vi "Deinitialize.vi"(8 "error in (no error)":errorcluster, 11 "IP Connection in":refnum<class "IP Connection.lvclass">) -> (0 "error out":errorcluster)   [LabVIEW 2011, in "Tinkerforge.lvlib" / "IP Connection.lvclass"]
doc: "This VI deinitializes the <B>IP Connection</B> class object and collects the called communication worker VI and disconnects from the Brickd."
uses:
  IP Connection.lvclass
  IP Connection.lvclass/IP Connection.ctl
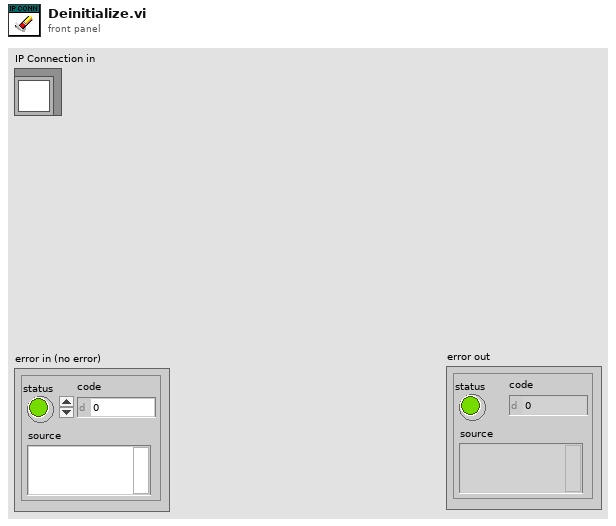
[diagram p1: front panel]
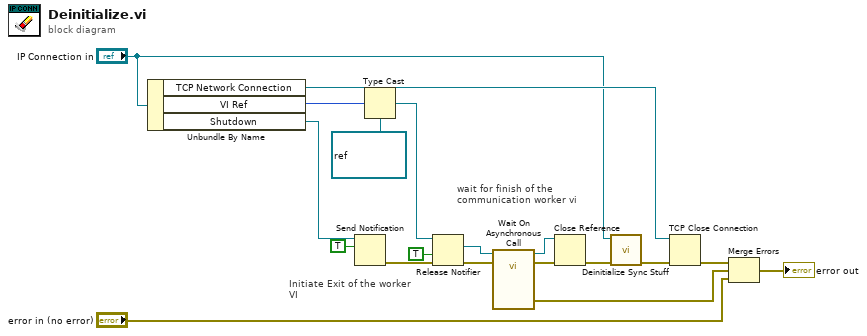
[diagram p0: block diagram]
diagram:
  # "Initiate Exit of the worker\nVI"
  # "wait for finish of the\ncommunication worker vi"
  n1 = Unbundle By Name("IP Connection in") -> ("TCP Network Connection"=w19:refnum<k5>, "VI Ref"=w18:u32, "Shutdown"=w2:refnum<notifier>)
  n2 = Send Notification(notification=TRUE, notifier=w2) -> (error out=w3:errorcluster)  [unwired: 1 in, 1 out]
  n3 = Type Cast(type=refnum<notifier> refnum ("notifier out"), x=w18) -> (*(type *) &x=w15:refnum<notifier>)
  n4 = Release Notifier(notifier=w15, force destroy? (F)=TRUE, error in (no error)=w3) -> (last notification=w14:refnum<vi>, error out=w16:errorcluster)  [unwired: 1 out]
  n5 = call-by-ref "Wait On Asynchronous Call"(reference=w14, error in=w16) -> (reference out=w11:refnum<vi>, error out=w12:errorcluster, 0:"error out"=w5:errorcluster)  [unwired: 10 in, 1 out]
  n6 = Close Reference(reference=w11, error in (no error)=w12) -> (error out=w9:errorcluster)
  n7 = call "Deinitialize Sync Stuff.vi"("error in (no error)"=w9, "IP Connection in"="IP Connection in") -> ("error out"=w8:errorcluster)  [unwired: 8 in, 1 out]
  n8 = TCP Close Connection(connection ID=w19, error in (no error)=w8) -> (error out=w6:errorcluster)  [unwired: 1 in, 1 out]
  n9 = Merge Errors(w6, w5, "error in (no error)") -> (→"error out":errorcluster)
